vi "W&R(Know Size CRC16 Without Data).vi"(0 "VISA resource name in":refnum<visa-resource-name>, 5 "写入指令/数据":string, 7 "总字节数":u32, 9 "超时":u32=1000, 11 "error in":errorcluster) -> (4 "VISA resource name out":refnum<visa-resource-name>, 15 "error out":errorcluster)   [LabVIEW 2018]
uses:
  <vilib>/Instr/_visa.llb/VISA Set IO Buffer Mask.ctl
  <vilib>/Instr/_visa.llb/VISA Flush IO Buffer Mask.ctl
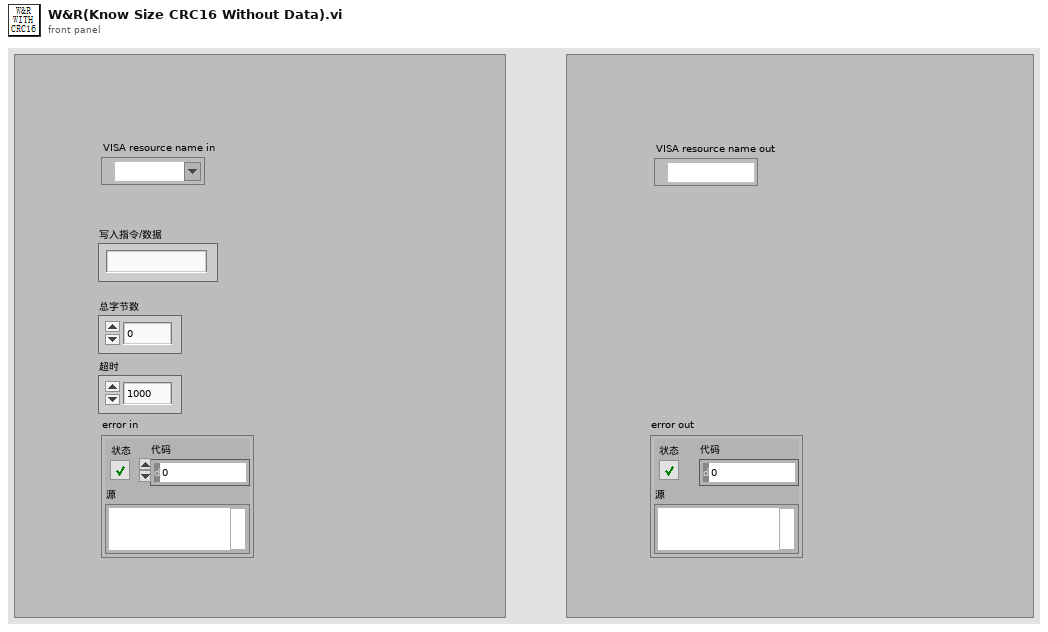
[diagram p1: front panel]
types:
  T1 = typedef "VISA Flush IO Buffer Mask.ctl" = u16
  T2 = typedef "VISA Set IO Buffer Mask.ctl" = u16
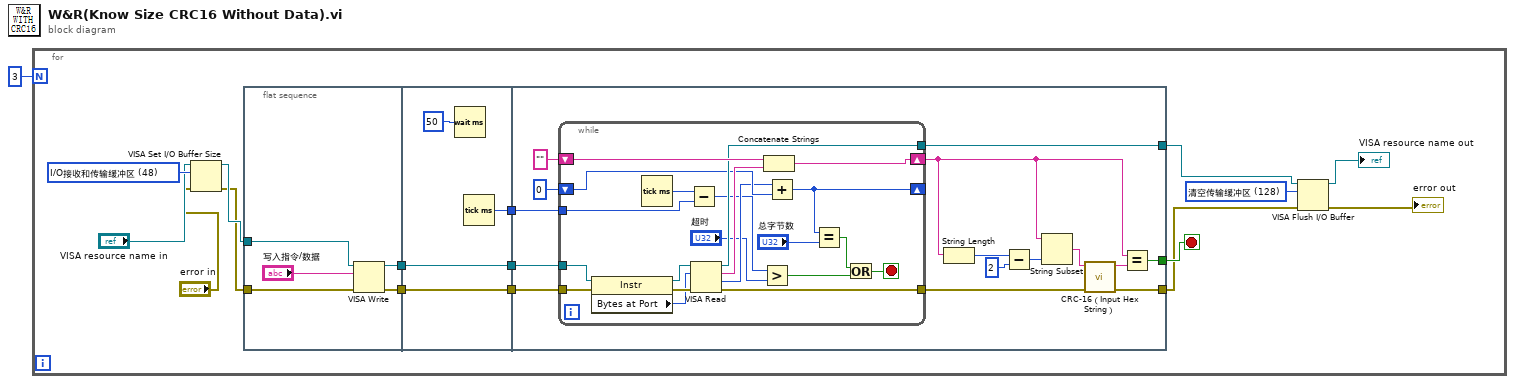
[diagram p0: block diagram]
diagram:
  n1 = for {
    N: 3 -> [_]
    stop <- w13 stop-if-true
    w6 = T1 128 items=["清空接收缓冲区"=16, "向设备写入传输缓冲区"=32, "清空接收缓冲区（无I/O）"=64, "清空传输缓冲区"=128] ("Mask")
    w11 = T2 48 items=["I/O接收缓冲区"=16, "I/O传输缓冲区"=32, "I/O接收和传输缓冲区"=48] ("Mask")
    n2 = VISA Set I/O Buffer Size(VISA resource name="VISA resource name in", mask (16)=w11, error in (no error)="error in") -> (VISA resource name out=w9:refnum<visa-resource-name>, error out=w7:errorcluster)  [unwired: 1 in]
    n3 = flat-sequence {
      tunnel: w9 -> [w22]
      tunnel: [w21] -> w17
      tunnel: [w19] -> w16
      tunnel: w7 -> [w18]
      tunnel: [w26] -> w15
      tunnel: w17 -> [w26]
      tunnel: [w25] -> w14
      tunnel: w16 -> [w25]
      tunnel: [w24] -> w12
      tunnel: w15 -> [w41]
      tunnel: w14 -> [w40]
      tunnel: [w35] -> w13
      tunnel: [w39] -> w5
      tunnel: [w27] -> w3
      tunnel: w12 -> [w36]
      frame #0 {
        n4 = VISA Write(VISA resource name=w22, write buffer="写入指令/数据", error in (no error)=w18) -> (VISA resource name out=w21:refnum<visa-resource-name>, error out=w19:errorcluster)  [unwired: 1 out]
      }
      frame #1 {
        n5 = Wait (ms)(milliseconds to wait=u32 50 ("等待时间（毫秒）")) -> ()  [unwired: 1 out]
        n6 = Tick Count (ms)() -> (millisecond timer value=w24:u32)
      }
      frame #2 {
        n7 = while {
          tunnel: w41 -> [w62]
          tunnel: w40 -> [w61]
          shift-right: [w58] -> w34
          shift-left: "" -> [w57]
          tunnel: [w56] -> w39
          tunnel: [w55] -> w28
          shift-right: [w51] -> _
          shift-left: u32 0 -> [w52]
          tunnel: w36 -> [w48]
          stop <- w44 stop-if-true
          n8 = property class="Instr"(reference=w62, error in=w61) -> (reference out=w60:refnum<visa-resource-name>, error out=w59:errorcluster, "Bytes at Port"=w53:u32)
          n9 = Tick Count (ms)() -> (millisecond timer value=w49:u32)
          n10 = Subtract(x=w49, y=w48) -> (x-y=w47:u32)
          n11 = VISA Read(VISA resource name=w60, byte count=w53, error in (no error)=w59) -> (VISA resource name out=w56:refnum<visa-resource-name>, read buffer=w54:string, return count=w50:u32, error out=w55:errorcluster)
          n12 = Greater?(x=w47, y="超时") -> (0:w45:bool)
          n13 = Concatenate Strings(w57, w54) -> (w58:string)
          n14 = Add(x=w50, y=w52) -> (x+y=w51:u32)
          n15 = Equal?(x=w51, y="总字节数") -> (x = y?=w46:bool)
          n16 = Or(x=w46, y=w45) -> (x .or. y?=w44:bool)
        }
        n17 = String Length(string=w34) -> (length=w33:i32)
        n18 = Subtract(x=w33, y=2) -> (x-y=w31:i32)
        n19 = String Subset(string=w34, length (rest)=w31) -> (substring=w30:string)  [unwired: 1 in]
        n20 = call "CRC-16（Input Hex String）.vi"("error in (no error)"=w28, "发送数据"=w30) -> ("error out"=w27:errorcluster, "完整命令"=w29:string)  [unwired: 8 in]
        n21 = Equal?(x=w34, y=w29) -> (x = y?=w35:bool)
      }
    }
    n22 = VISA Flush I/O Buffer(VISA resource name=w5, mask (16)=w6, error in (no error)=w3) -> (VISA resource name out=→"VISA resource name out":refnum<visa-resource-name>, error out=→"error out":errorcluster)
  }
